vi "核查数据断电保存 (子VI).vi"   [LabVIEW 2016, in "数据传输系统-04.lvlib"]
uses:
  <vilib>/Utility/config.llb/NI_LVConfig.lvlib
types:
  T1 = cluster{"setini":string, "sysini":string, "hechaini":string, "actualwrite":string, "actualread":string, "datasent":string, "反控命令信息队列":string, "反控与仪器交互":string}
  T2 = typedef "NI_LVConfig.lvlib/Config Data RefNum.ctl" = refnum<k1>
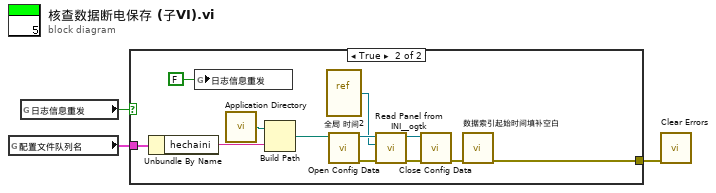
[diagram p0: block diagram]
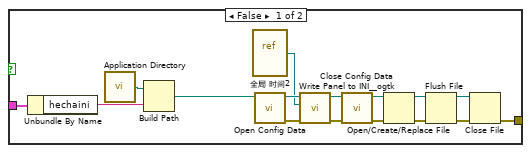
[diagram p2: hidden frame]
diagram:
  n1 = global read "全局1.vi" "配置文件队列名"() -> (w2:T1)
  n2 = global read "断电保存全局.vi" "日志信息重发"() -> (w3:bool)
  n3 = case shown="True" w3 {
    tunnel: w2 -> [w5 w21]
    tunnel: [w4 w20] -> w1
    frame False {
      n4 = Unbundle By Name(w5) -> ("hechaini"=w6:string)
      n5 = call <vilib>:"Application Directory.vi"() -> ("Application Directory"=w7:path)
      n6 = Build Path(base path=w7, name or relative path=w6) -> (appended path=w8:path)
      n7 = vi-ref "全局 时间2.vi"() -> (w9:refnum<vi>)
      n8 = call <vilib>:"Open Config Data.vi"("configuration file path"=w8) -> ("error out"=w11:errorcluster, "refnum"=w19:T2)  [unwired: 8 in, 1 out]
      n9 = call <userlib>:"Write Panel to INI__ogtk.vi"("error in (no error)"=w11, "VI ref"=w9, "refnum"=w19) -> ("error out"=w12:errorcluster, "refnum out"=w10:T2)  [unwired: 7 in]
      n10 = call <vilib>:"Close Config Data.vi"("error in (no error)"=w12, "refnum"=w10) -> ("error out"=w17:errorcluster, "file path"=w18:path)  [unwired: 8 in]
      n11 = Open/Create/Replace File(file path (use dialog)=w18, error in=w17) -> (refnum out=w14:refnum<file>, error out=w13:errorcluster)  [unwired: 4 in, 1 out]
      n12 = Flush File(refnum=w14, error in=w13) -> (refnum out=w15:refnum<file>, error out=w16:errorcluster)
      n13 = Close File(refnum=w15, error in=w16) -> (error out=w4:errorcluster)  [unwired: 1 out]
    }
    frame True {
      n14 = Unbundle By Name(w21) -> ("hechaini"=w30:string)
      n15 = global write "断电保存全局.vi" "日志信息重发"(FALSE ("日志信息重发")) -> ()
      n16 = call <vilib>:"Application Directory.vi"() -> ("Application Directory"=w23:path)
      n17 = Build Path(base path=w23, name or relative path=w30) -> (appended path=w22:path)
      n18 = vi-ref "全局 时间2.vi"() -> (w25:refnum<vi>)
      n19 = call <vilib>:"Open Config Data.vi"("configuration file path"=w22) -> ("error out"=w27:errorcluster, "refnum"=w26:T2)  [unwired: 8 in, 1 out]
      n20 = call <userlib>:"Read Panel from INI__ogtk.vi"("error in (no error)"=w27, "VI ref"=w25, "refnum"=w26) -> ("error out"=w28:errorcluster, "refnum out"=w24:T2)  [unwired: 7 in]
      n21 = call <vilib>:"Close Config Data.vi"("error in (no error)"=w28, "refnum"=w24) -> ("error out"=w29:errorcluster)  [unwired: 8 in, 1 out]
      n22 = call "数据索引起始时间填补空白.vi"("error in (no error)"=w29) -> ("error out"=w20:errorcluster)  [unwired: 10 in]
    }
  }
  n23 = call <vilib>:"Clear Errors.vi"("error in (no error)"=w1) -> ()  [unwired: 5 in, 2 out]
